vi "myRIO_emulated.vi"() -> ()   [LabVIEW 2017]
uses:
  <vilib>/NI/STM/SubVIs/MetaDataElement.ctl
  <vilib>/NI/STM/TCP/TCP Read Options.ctl
  <vilib>/NI/STM/TCP/Write Meta Data (TCP Ref).vi
  <vilib>/NI/STM/TCP/Get Connection Reference (TCP).vi
  <vilib>/NI/STM/TCP/Write Meta Data (TCP Clst).vi
  <vilib>/NI/STM/TCP/Read Message (TCP).vi
  <vilib>/NI/STM/TCP/Write Message (TCP).vi
  <vilib>/NI/STM/NI STM.lvlib
panel:
  in  "stop":bool
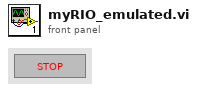
[diagram p1: front panel]
types:
  T1 = typedef "NI STM.lvlib/MetaDataElement.ctl" = string
  T2 = typedef "NI STM.lvlib/TCP Connection Info.ctl" = cluster{"connection ID":refnum<k5>, "meta data":T1[]}
  T3 = typedef "NI STM.lvlib/TCP Read Options.ctl" = cluster{"ignore timeout error":bool, "timeout ms (1000)":i32}
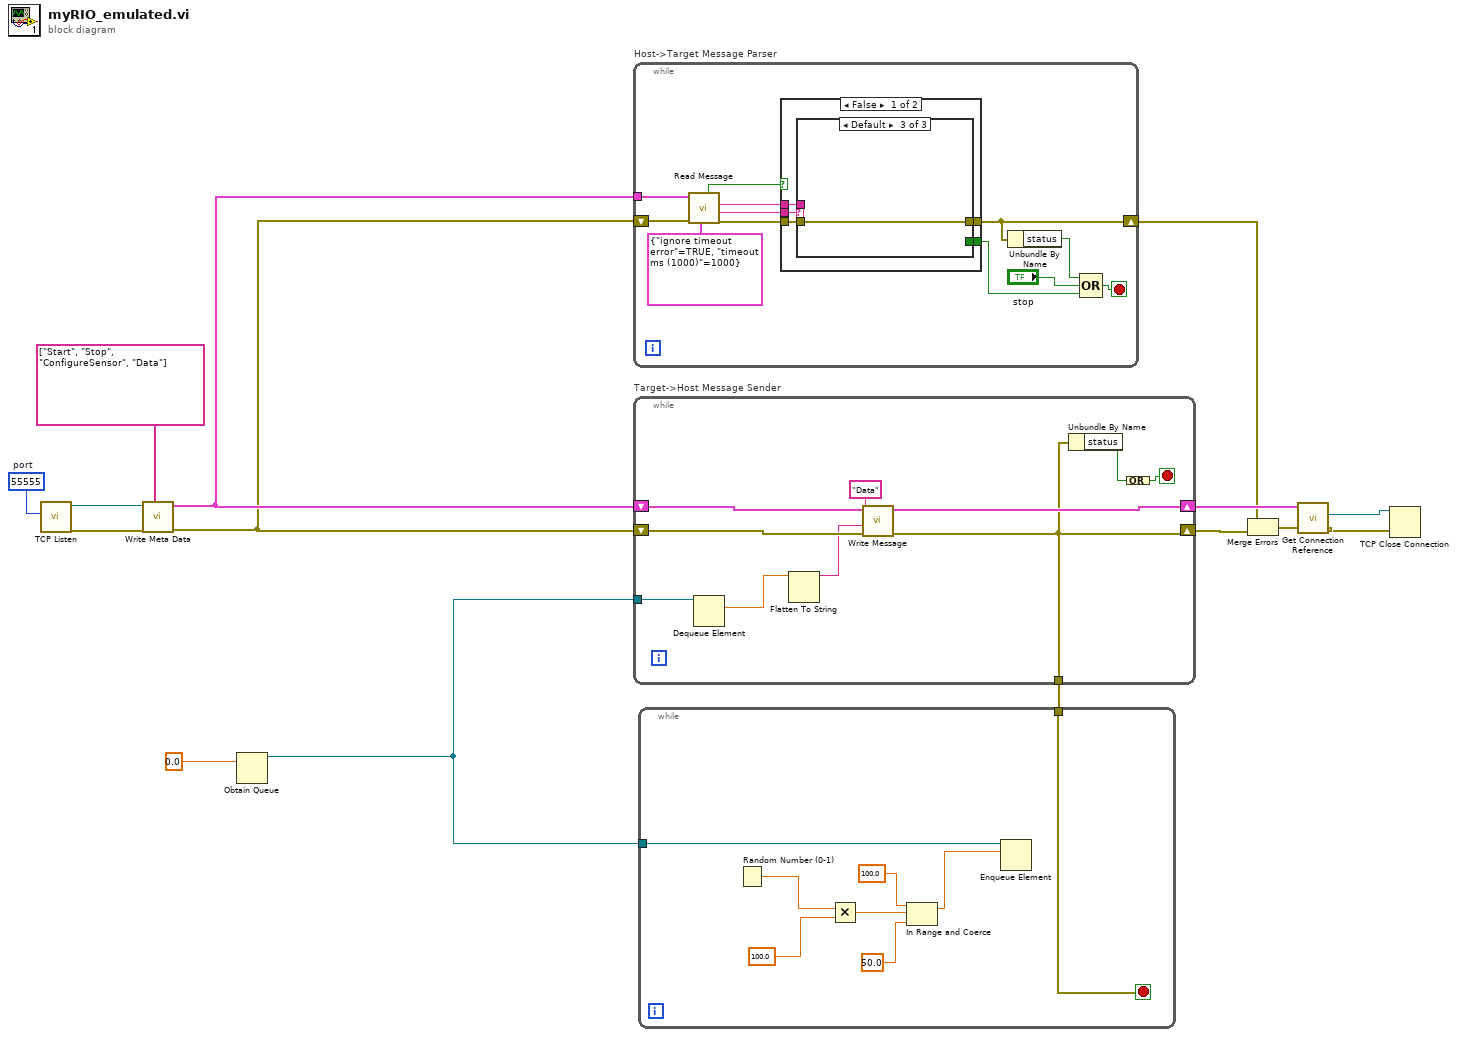
[diagram p0: block diagram]
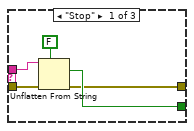
[diagram p2: hidden frame]
diagram:
  w15 = u16 55555  # port
  n1 = call <vilib>:"TCP Listen.vi"("port"=w15) -> ("error out"=w13:errorcluster, "connection ID"=w14:refnum<k5>)  [unwired: 3 in, 6 out]
  n2 = call-poly <vilib>:"Write Meta Data.vi"("meta data"=T1[] ["Start", "Stop", "ConfigureSensor", "Data"], "error in"=w13, "connection ID"=w14) -> ("error out"=w11:errorcluster, "connection info out"=w12:T2)  [unwired: 2 in, 5 out]
  n3 = Obtain Queue(element data type=0.0) -> (queue out=w3:refnum<queue>)  [unwired: 4 in, 2 out]
  n4 = while "Host->Target Message Parser" {
    tunnel: w12 -> [w27]
    shift-right: [w20] -> w7
    shift-left: w11 -> [w26]
    stop <- w17 stop-if-true
    n5 = call-poly <vilib>:"Read Message.vi"("options"=T3 {"ignore timeout error"=TRUE, "timeout ms (1000)"=1000} ("Options"), "error in"=w26, "connection info in"=w27) -> ("error out"=w22:errorcluster, "name"=w25:T1, "data string"=w24:string, "timed out?"=w23:bool)  [unwired: 2 in, 3 out]
    n6 = case shown="False" w23 {
      tunnel: w25 -> [w29 _]
      tunnel: w24 -> [w32 _]
      tunnel: w22 -> [w31 w40]
      tunnel: [w30 w40] -> w20
      tunnel: [w28 _] -> w16
      frame False {
        n7 = case shown="Default" w29 {
          tunnel: w32 -> [w36 _ _]
          tunnel: w31 -> [w35 w38 w39]
          tunnel: [w33 w38 w39] -> w30
          tunnel: [w34 _ _] -> w28
          frame "Stop" {
            n8 = Unflatten From String(type=FALSE, binary string=w36, error in (no error)=w35) -> (value=w34:bool, error out=w33:errorcluster)  [unwired: 1 in, 2 out]
          }
          frame "Start" {
          }
          frame Default {
          }
        }
      }
      frame True {
      }
    }
    n9 = Unbundle By Name(w20) -> ("status"=w19:bool)
    n10 = Compound Arithmetic op=OR(w19, "stop", w16) -> (w17:bool)
  }
  n11 = while "Target->Host Message Sender" {
    shift-right: [w41] -> w8
    shift-left: w11 -> [w46]
    shift-right: [w49] -> w10
    shift-left: w12 -> [w50]
    tunnel: w3 -> [w44]
    tunnel: [w41] -> w1
    stop <- w47 stop-if-true
    n12 = Dequeue Element(queue=w44) -> (element=w43:dbl)  [unwired: 2 in, 3 out]
    n13 = Flatten To String(anything=w43) -> (data string=w42:string)  [unwired: 3 in, 2 out]
    n14 = call-poly <vilib>:"Write Message.vi"("error in"=w46, "data"=w42, "name"="Data" ("Name"), "connection info in"=w50) -> ("error out"=w41:errorcluster, "connection info out"=w49:T2)  [unwired: 1 in, 5 out]
    n15 = Unbundle By Name(w41) -> ("status"=w48:bool)
    n16 = Compound Arithmetic op=OR(w48) -> (w47:bool)
  }
  n17 = while {
    tunnel: w3 -> [w52]
    tunnel: w1 -> [w51]
    stop <- w51 stop-if-true
    n18 = Random Number (0-1)() -> (number: 0 to 1=w57:dbl)
    n19 = Multiply(x=w57, y=100.0) -> (x*y=w56:dbl)
    n20 = In Range and Coerce(upper limit=100.0, x=w56, lower limit=50.0) -> (coerced(x)=w53:dbl)  [unwired: 1 out]
    n21 = Enqueue Element(queue=w52, element=w53) -> ()  [unwired: 2 in, 3 out]
  }
  n22 = Merge Errors(w7, w8) -> (w6:errorcluster)
  n23 = call-poly <vilib>:"Get Connection Reference.vi"("error in"=w6, "connection info in"=w10) -> ("error out"=w4:errorcluster, "connection ID out"=w9:refnum<k5>)  [unwired: 8 out]
  n24 = TCP Close Connection(connection ID=w9, error in (no error)=w4) -> ()  [unwired: 3 out]
